vi "err p.vi"(7 "err":bool) -> (8 "p":dbl)   [LabVIEW 2017]
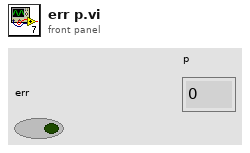
[diagram p1: front panel]
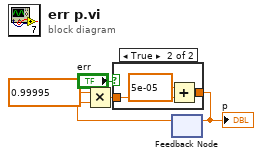
[diagram p0: block diagram]
diagram:
  n1 = feedback #1() -> (w3:dbl)  [unwired: 1 in]
  n2 = Multiply(x=0.99995, y=w3) -> (x*y=w4:dbl)
  n3 = case shown="True" "err" {
    tunnel: [w6 w8] -> w5
    tunnel: w4 -> [w6 w7]
    frame False {
    }
    frame True {
      n4 = Add(x=5e-05, y=w7) -> (x+y=w8:dbl)
    }
  }
  "p" <- w5
  n5 = feedback-in #1(w5) -> ()
